vi "File.Copy Source Dir to Targert Dir, Only Newer Files.vi"(9 "Do Not Overwrite if Exists":bool, 10 "Target Dir":path, 11 "Source Dir":path) -> (0 "Error Out":errorcluster, 3 "Copied Files":path[](array[path]))   [LabVIEW 2024]
uses:
  File Utils.lvlib
panel:
  in  "error in (no error)":errorcluster
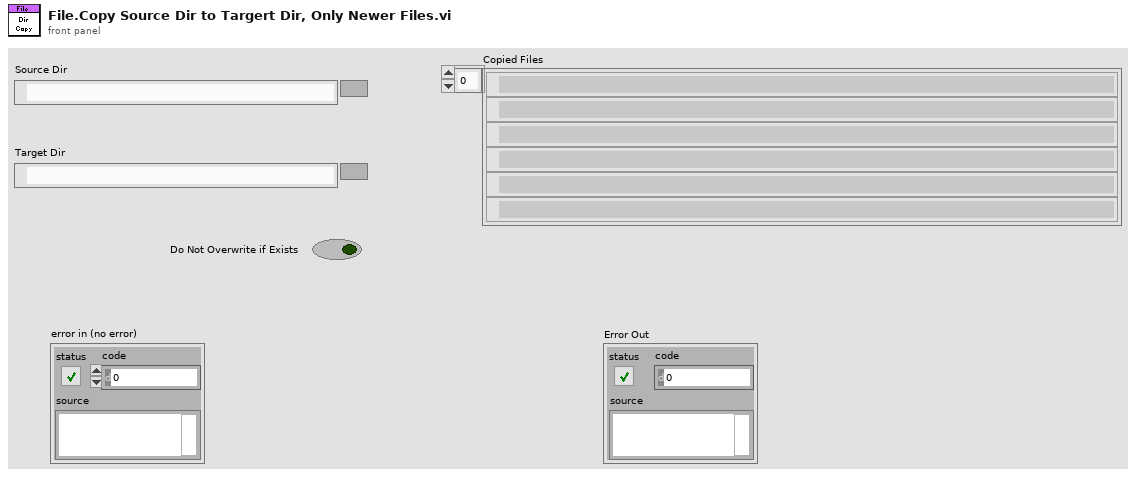
[diagram p1: front panel]
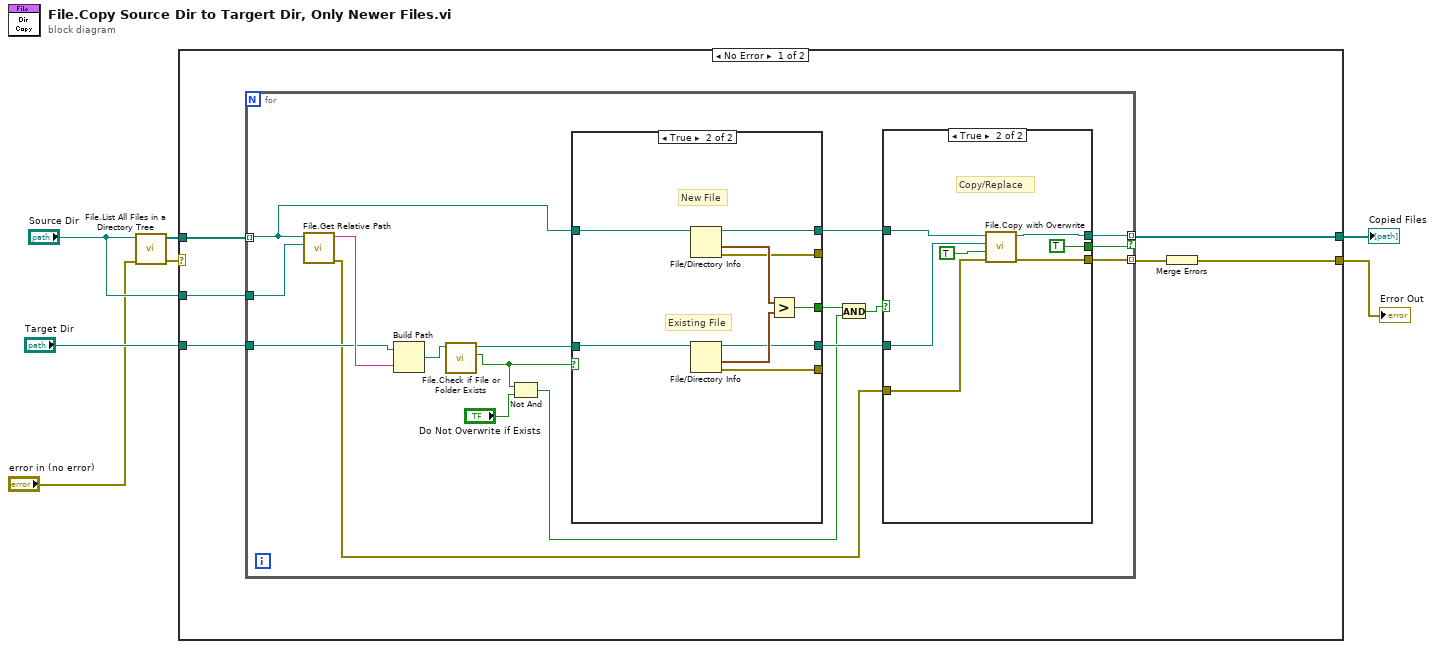
[diagram p0: block diagram]
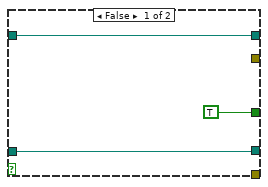
[diagram p3: hidden frame]
diagram:
  n1 = call "File.List All Files in a Directory Tree.vi"("error in (no error)"="error in (no error)", "Folder"="Source Dir") -> ("error out"=w4:errorcluster, "Files"=w7:path[])  [unwired: 8 in]
  n2 = case shown="No Error" w4 {
    selector: w4 -> [_ w50]
    tunnel: w7 -> [w13 _]
    tunnel: "Source Dir" -> [w12 _]
    tunnel: "Target Dir" -> [w11 _]
    tunnel: [w9 w50] -> w2
    tunnel: [w8 _] -> w3
    frame No Error {
      n3 = for {
        tunnel: w13 -> [w27] mode=indexing
        tunnel: w12 -> [w30]
        tunnel: w11 -> [w28]
        tunnel: [w22] -> w10 mode=indexing
        tunnel: [w21] -> w8 mode=indexing if=w20
        n4 = call "File.Get Relative Path.vi"("Root Dir"=w30, "Path"=w27) -> ("error out"=w19:errorcluster, "Relative Path"=w29:string)  [unwired: 8 in]
        n5 = Build Path(base path=w28, name or relative path=w29) -> (appended path=w26:path)
        n6 = call "File.Check if File or Folder Exists.vi"("Path"=w26) -> ("Exists"=w18:bool, "Dup Path"=w25:path)  [unwired: 6 in, 3 out]
        n7 = Not And(1:"Do Not Overwrite if Exists", 2:w18) -> (0:w14:bool)
        n8 = case shown="True" w18 {
          tunnel: w27 -> [w39 w49]
          tunnel: w25 -> [w38 w48]
          tunnel: [TRUE w45] -> w16
          tunnel: [w39 w44] -> w24
          tunnel: [w38 w43] -> w23
          tunnel: [_ w42] -> _
          tunnel: [_ w41] -> _
          frame False {
          }
          frame True {
            # "Existing File"
            # "New File"
            n9 = File/Directory Info(path=w49) -> (path out=w44:path, last mod=w47:timestamp, error out=w41:errorcluster)  [unwired: 1 in, 4 out]
            n10 = File/Directory Info(path=w48) -> (path out=w43:path, last mod=w46:timestamp, error out=w42:errorcluster)  [unwired: 1 in, 4 out]
            n11 = Greater?(x=w47, y=w46) -> (0:w45:bool)
          }
        }
        n12 = And(x=w16, y=w14) -> (x .and. y?=w15:bool)
        n13 = case shown="True" w15 {
          tunnel: w24 -> [_ w37]
          tunnel: w23 -> [_ w36]
          tunnel: [_ w35] -> w22
          tunnel: [_ w33] -> w21
          tunnel: [_ TRUE] -> w20
          tunnel: w19 -> [_ w32]
          frame False {
            # "Ignore"
          }
          frame True {
            # "Copy/Replace"
            n14 = call "File.Copy with Overwrite.vi"("error in (no error)"=w32, "Dest is Dir(F)/File(T)"=TRUE, "Destination"=w36, "Source"=w37) -> ("error out"=w35:errorcluster, "Destination Dup"=w33:path)  [unwired: 5 in, 1 out]
          }
        }
      }
      n15 = Merge Errors(w10) -> (w9:errorcluster)
    }
    frame Error {
    }
  }
  "Copied Files" <- w3
  "Error Out" <- w2
